vi "Log Configuration.vi"(8 "error in (no error)":errorcluster, 10 "Enum":enum16{"System", "Devices", "AO", "AI", "MCLI"}(ring), 11 "Instrument.Lockin in":refnum<class "Instrument.Lockin.lvclass">) -> (0 "error out":errorcluster, 3 "Instrument.Lockin out":refnum<class "Instrument.Lockin.lvclass">)   [LabVIEW 2019, in "Instrument.Lockin.lvlib" / "Instrument.Lockin.lvclass"]
uses:
  Instrument.Lockin.lvclass
  C:/Program Files (x86)/National Instruments/LabVIEW 2019/user.lib/LevyLab/Instrument Framework/Instrument/Instrument.lvclass
  <userlib>/LevyLab/Instrument Framework/Instrument/Instrument.lvclass
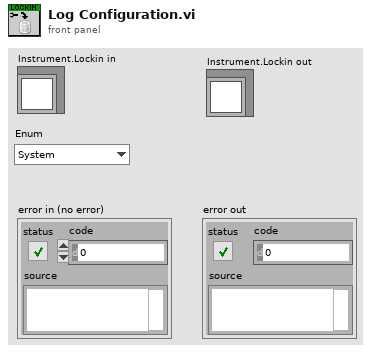
[diagram p1: front panel]
types:
  T1 = typedef "Instrument.Lockin.lvlib/Instrument.Lockin.lvclass/Lockin.LogConfiguration.System--Cluster.ctl" = cluster{"System Serial Number":string, "Chassis Serial Number":string, "Chassis Type":string, "Sample Rate":dbl}
  T2 = typedef "Instrument.Lockin.lvlib/Instrument.Lockin.lvclass/Lockin.LogConfiguration.Devices--Cluster.ctl" = cluster{"System Serial Number":string, "Chassis Serial Number":string, "Device Serial Number":string, "Device Type":string, "Chassis Slot":i32, "Device Temperature":dbl, "Device Calibration Temperature":dbl, "Device Calibration Time":string}
  T3 = typedef "Instrument.Lockin.lvlib/Instrument.Lockin.lvclass/Lockin.LogConfiguration.Channels--Cluster.ctl" = cluster{"System Serial Number":string, "System Channel":i32, "Device Serial Number":string, "Device Channel":i32, "Channel Type":string, "Channel Coupling":string, "Channel Range":string, "Channel Configuration":string}
  T4 = typedef "Instrument.Lockin.lvlib/Instrument.Lockin.lvclass/Lockin.LogConfiguration.MCLI--Cluster.ctl" = cluster{"System Serial Number":string, "Software Version":string, "REF Channel":i32, "frequency":dbl, "time constant":dbl, "roll-off":i32}
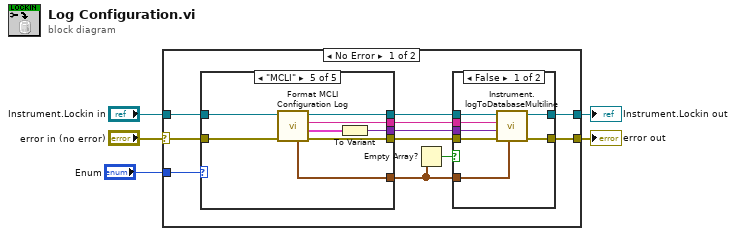
[diagram p0: block diagram]
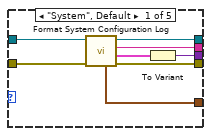
[diagram p2: hidden frame]
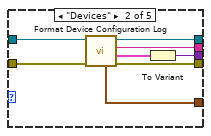
[diagram p3: hidden frame]
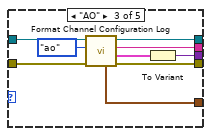
[diagram p4: hidden frame]
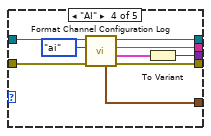
[diagram p5: hidden frame]
diagram:
  n1 = case shown="No Error" "error in (no error)" {
    selector: "error in (no error)" -> [w7 w69]
    tunnel: "Instrument.Lockin in" -> [w12 w68]
    tunnel: [w15 w69] -> w4
    tunnel: [w16 w68] -> w2
    tunnel: "Enum" -> [w13 _]
    frame No Error {
      n2 = case shown="\"MCLI\"" w13 {
        tunnel: w12 -> [w24 w32 w41 w50 w58]
        tunnel: [w23 w31 w40 w49 w57] -> w11
        tunnel: [w22 w30 w39 w48 w56] -> w10
        tunnel: [w20 w28 w37 w46 w54] -> w9
        tunnel: [w19 w27 w36 w45 w53] -> w8
        tunnel: w7 -> [w18 w26 w35 w44 w52]
        tunnel: [w17 w25 w34 w43 w51] -> w6
        frame "System", Default {
          n3 = call "Format System Configuration Log.vi"("error in (no error)"=w18, "Instrument.Lockin in"=w24) -> ("error out"=w19:errorcluster, "System Configuration"=w21:T1[], "Paths"=w22:string, "Instrument.Lockin out"=w23:refnum<class "Instrument.Lockin.lvclass">, "Times"=w17:timestamp[])  [unwired: 5 in]
          n4 = To Variant(anything=w21) -> (Variant=w20:variant)
        }
        frame "Devices" {
          n5 = call "Format Device Configuration Log.vi"("error in (no error)"=w26, "Instrument.Lockin in"=w32) -> ("error out"=w27:errorcluster, "Device Configuration"=w29:T2[], "Log Paths"=w30:string, "Instrument.Lockin out"=w31:refnum<class "Instrument.Lockin.lvclass">, "Times"=w25:timestamp[])  [unwired: 5 in]
          n6 = To Variant(anything=w29) -> (Variant=w28:variant)
        }
        frame "AO" {
          n7 = call "Format Channel Configuration Log.vi"("error in (no error)"=w35, "Channel Type (ao/ai)"=enum16{"ao", "ai"}."ao", "Instrument.Lockin in"=w41) -> ("error out"=w36:errorcluster, "Channel Configuration"=w38:T3[], "Log Paths"=w39:string, "Instrument.Lockin out"=w40:refnum<class "Instrument.Lockin.lvclass">, "Times"=w34:timestamp[])  [unwired: 4 in]
          n8 = To Variant(anything=w38) -> (Variant=w37:variant)
        }
        frame "AI" {
          n9 = call "Format Channel Configuration Log.vi"("error in (no error)"=w44, "Channel Type (ao/ai)"=enum16{"ao", "ai"}."ai", "Instrument.Lockin in"=w50) -> ("error out"=w45:errorcluster, "Channel Configuration"=w47:T3[], "Log Paths"=w48:string, "Instrument.Lockin out"=w49:refnum<class "Instrument.Lockin.lvclass">, "Times"=w43:timestamp[])  [unwired: 4 in]
          n10 = To Variant(anything=w47) -> (Variant=w46:variant)
        }
        frame "MCLI" {
          n11 = call "Format MCLI Configuration Log.vi"("error in (no error)"=w52, "Instrument.Lockin in"=w58) -> ("error out"=w53:errorcluster, "Log Data"=w55:T4[], "Log Paths"=w56:string, "Instrument.Lockin out"=w57:refnum<class "Instrument.Lockin.lvclass">, "Times"=w51:timestamp[])  [unwired: 5 in]
          n12 = To Variant(anything=w55) -> (Variant=w54:variant)
        }
      }
      n13 = Empty Array?(array=w6) -> (empty?=w14:bool)
      n14 = case shown="False" w14 {
        tunnel: [w65 w66] -> w15
        tunnel: [w64 w67] -> w16
        tunnel: w11 -> [w63 w67]
        tunnel: w10 -> [w62 _]
        tunnel: w9 -> [w61 _]
        tunnel: w8 -> [w60 w66]
        tunnel: w6 -> [w59 _]
        frame False {
          n15 = call <userlib>:"Instrument.logToDatabaseMultiline.vi"("timestamps"=w59, "error in (no error)"=w60, "Data"=w61, "Paths"=w62, "Instrument"=w63) -> ("error out"=w65:errorcluster, "Instrument out"=w64:refnum<class "Instrument.Lockin.lvclass">)  [unwired: 5 in]
        }
        frame True {
        }
      }
    }
    frame Error {
    }
  }
  "error out" <- w4
  "Instrument.Lockin out" <- w2
